vi "Test Get Wire Data Type.vi"() -> ()   [LabVIEW 2014]
uses:
  <vilib>/Utility/VariantDataType/Type.ctl
  <vilib>/fxp/LVFixedPointRepBitsTypeDef.ctl
  <vilib>/Utility/VariantDataType/VariantType.lvlib
panel:
  out "call chain":string[](array[string])
  out "FxpRepresentation":T1
  out "VI control datatypes":T2[](array[typedef])
  in  "vi path":path=path "C:/Users/lubo/Documents/LabView/LabVIEW-Universal-Transcriptor/Test/Examples For Parsing/Some VI.vi"
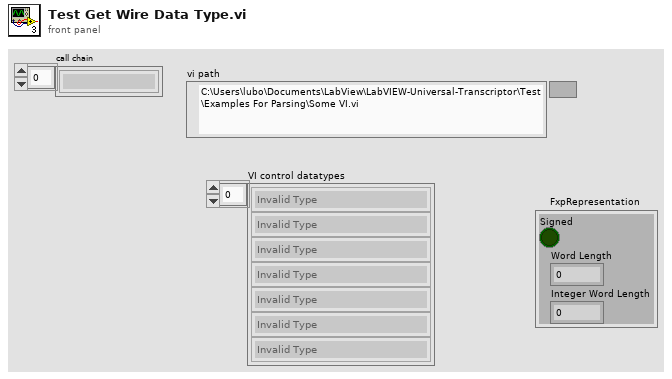
[diagram p1: front panel]
types:
  T1 = typedef "LVFixedPointRepBitsTypeDef.ctl" = cluster{"Signed":bool, "Word Length":u32, "Integer Word Length":i32}
  T2 = typedef "VariantType.lvlib/Type.ctl" = enum8{"Invalid Type", "Void", "I8", "I16", "I32", "I64", "U8", "U16", "U32", "U64", "Single Float", "Double Float", "Extended Float", "Single Complex", "Double Complex", "Extended Complex", "Enum U8", "Enum U16", "Enum U32", "Enum U64", "Single Float With Unit", "Double Float With Unit", "Extended Float With Unit", "Single Complex with Unit", "Double Complex with Unit", "Extended Complex with Unit", "Boolean", "String", "Path", "Picture", "Tag", "Array", "Cluster", "Variant", "LV Variant", "Waveform", "Timestamp", "Digital Waveform", "Digital Data", "ExpressData", "Refnum", "External Data", "VI", "Poly VI", "LabVIEW Class Instance", "Fixed Point"}
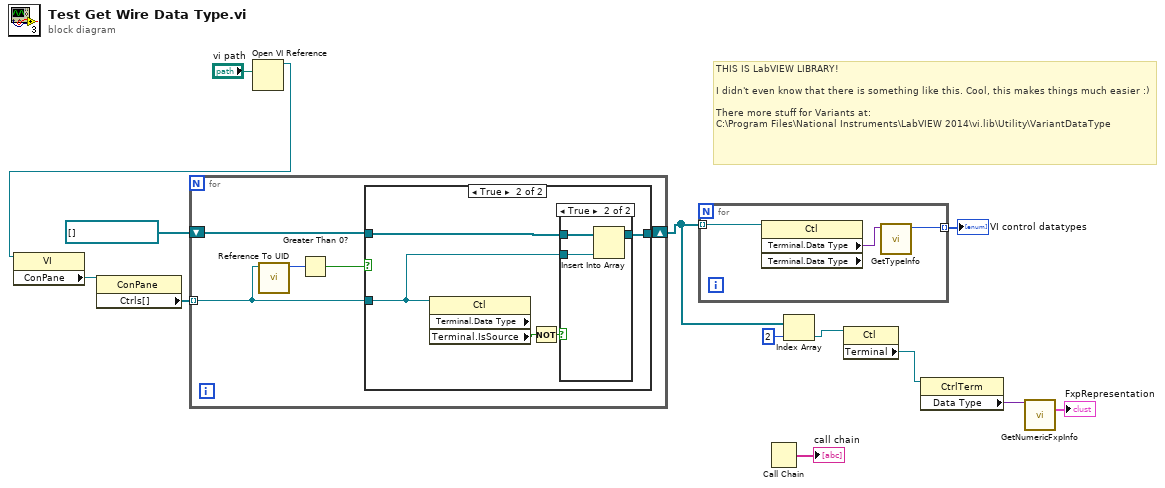
[diagram p0: block diagram]
diagram:
  # "THIS IS LabVIEW LIBRARY!\n\nI didn't even know that there is something like this. Cool, this makes things much easier :)\n\nThere more stuff for Variants at:\nC:\\Program Files\\National Instruments\\LabVIEW 2014\\vi.lib\\Utility\\VariantDataType"
  n1 = Open VI Reference(vi path="vi path") -> (vi reference=w9:refnum<vi>)  [unwired: 5 in, 1 out]
  n2 = property class="VI"(reference=w9) -> ("ConPane"=w12:refnum<vi>)  [unwired: 1 in, 2 out]
  n3 = property class="ConPane"(reference=w12) -> ("Ctrls[]"=w11:refnum<vi>[])  [unwired: 1 in, 2 out]
  n4 = for {
    tunnel: w11 -> [w16] mode=indexing
    shift-right: [w17] -> w7
    shift-left: refnum<vi>[] [] -> [w18]
    n5 = call "Reference To UID.vi"("Reference"=w16) -> ("UID"=w15:i32)  [unwired: 10 in]
    n6 = Greater Than 0?(x=w15) -> (x > 0?=w14:bool)
    n7 = case shown="True" w14 {
      tunnel: w18 -> [w19 w24]
      tunnel: w16 -> [_ w23]
      tunnel: [w19 w22] -> w17
      frame False {
      }
      frame True {
        n8 = property class="Ctl" props=["Terminal", "Data Type", "Terminal", "IsSource"](reference=w23) -> ("Terminal.IsSource"=w21:bool)  [unwired: 1 in, 3 out]
        n9 = Not(x=w21) -> (.not. x?=w20:bool)
        n10 = case shown="True" w20 {
          tunnel: w24 -> [w25 w28]
          tunnel: w23 -> [_ w27]
          tunnel: [w25 w26] -> w22
          frame False {
          }
          frame True {
            n11 = Insert Into Array(array=w28, new element=w27) -> (w26:refnum<vi>[])  [unwired: 1 in]
          }
        }
      }
    }
  }
  n12 = for {
    tunnel: w7 -> [w31] mode=indexing
    tunnel: [w29] -> w8 mode=indexing
    n13 = property class="Ctl" props=["Terminal", "Data Type", "Terminal", "Data Type"](reference=w31) -> ("Terminal.Data Type"=w30:variant)  [unwired: 1 in, 3 out]
    n14 = call <vilib>:"GetTypeInfo.vi"("Variant"=w30) -> ("Type Enum"=w29:T2)  [unwired: 6 in, 4 out]
  }
  "VI control datatypes" <- w8
  n15 = Call Chain() -> (call chain=→"call chain":string[])
  n16 = Index Array(array=w7, index=2) -> (element=w5:refnum<vi>)
  n17 = property class="Ctl"(reference=w5) -> ("Terminal"=w4:refnum<vi>)  [unwired: 1 in, 2 out]
  n18 = property class="CtrlTerm"(reference=w4) -> ("Data Type"=w3:variant)  [unwired: 1 in, 2 out]
  n19 = call <vilib>:"GetNumericFxpInfo.vi"("Variant"=w3) -> ("FxpRepresentation"=→"FxpRepresentation":T1)  [unwired: 10 in, 4 out]
